vi "Outline_Station.vi"(8 "error in (no error)":errorcluster, 11 "Main":T1={"Tite"="", "Base path"=path "", "Table"=[], "Stations"=[], "Shield Array"=[], "UPHs"=[], "VISA"={"VISA"="", "baud rate"=9600, "data bits"=8, "parity"=enum."None", "stop bits"=10, "flow control"=0}, "Path"={"roof"=path "", "Config"=path "", "Png"=path ""}, "Ctr"={"DB Dispaly"=refnum, "Error Table"=refnum, "Display"=refnum, "Login"=refnum, "Exit"=refnum, "FTT_Submit"=refnum}, "Login"={"User"="", "Grade"=""}, "information"={"cause"="", "Type"=enum."Inform", "code"=0, "Suroce"="", "Status"=FALSE}, "Local DB"={"Connstr"="", "Database"={"Constr"={"Driver"="", "Server"="", "User"="", "Pwd"="", "Database"=""}, "conn ref"=refnum, "State"=FALSE}}, "Remote DB"={"Connstr"="", "Database"={"Constr"={"Driver"="", "Server"="", "User"="", "Pwd"="", "Database"=""}, "conn ref"=refnum, "State"=FALSE}}, "FTT TV"="", "ExchangeTime"=0, "NVH"="", "EOL Path"=path ""} {"VISA"."flow control" items=["None", "XON/XOFF", "RTS/CTS", "XON/XOFF & RTS/CTS", "DTR/DSR", "XON/XOFF & DTR/DSR"]; "VISA"."stop bits" items=["1.0"=10, "1.5"=15, "2.0"=20]}) -> (0 "error out":errorcluster)   [LabVIEW 2014]
uses:
  Type'def/Online_Table.ctl
  Simatic S7/Function/Read/Read Sigle Data/Read Sigle Bool.vi
  <vilib>/ptbypt/NI_PtbyPt.lvlib
  Simatic S7/Function/Read/Read Sigle Data/Read Sigle String.vi
  <vilib>/addons/database/_DB Variant To Data/Database Variant To Data.xnode
  Type'def/FTT Display Type.ctl
  Type'def/UPH Config.ctl
  VISA/Ctr/VISA Ctr.ctl
  Type'def/Main Ctr Ref.ctl
  Type'def/User Login.ctl
  Database/Ctr/Constr.ctl
  <vilib>/addons/database/Connection.llb/Conn ObjectReference.ctl
  <vilib>/addons/database/NI_Database_API.lvlib
  Database/Ctr/Conneect State.ctl
  Type'def/MainCtr.ctl
panel:
  in  "Boolean":bool
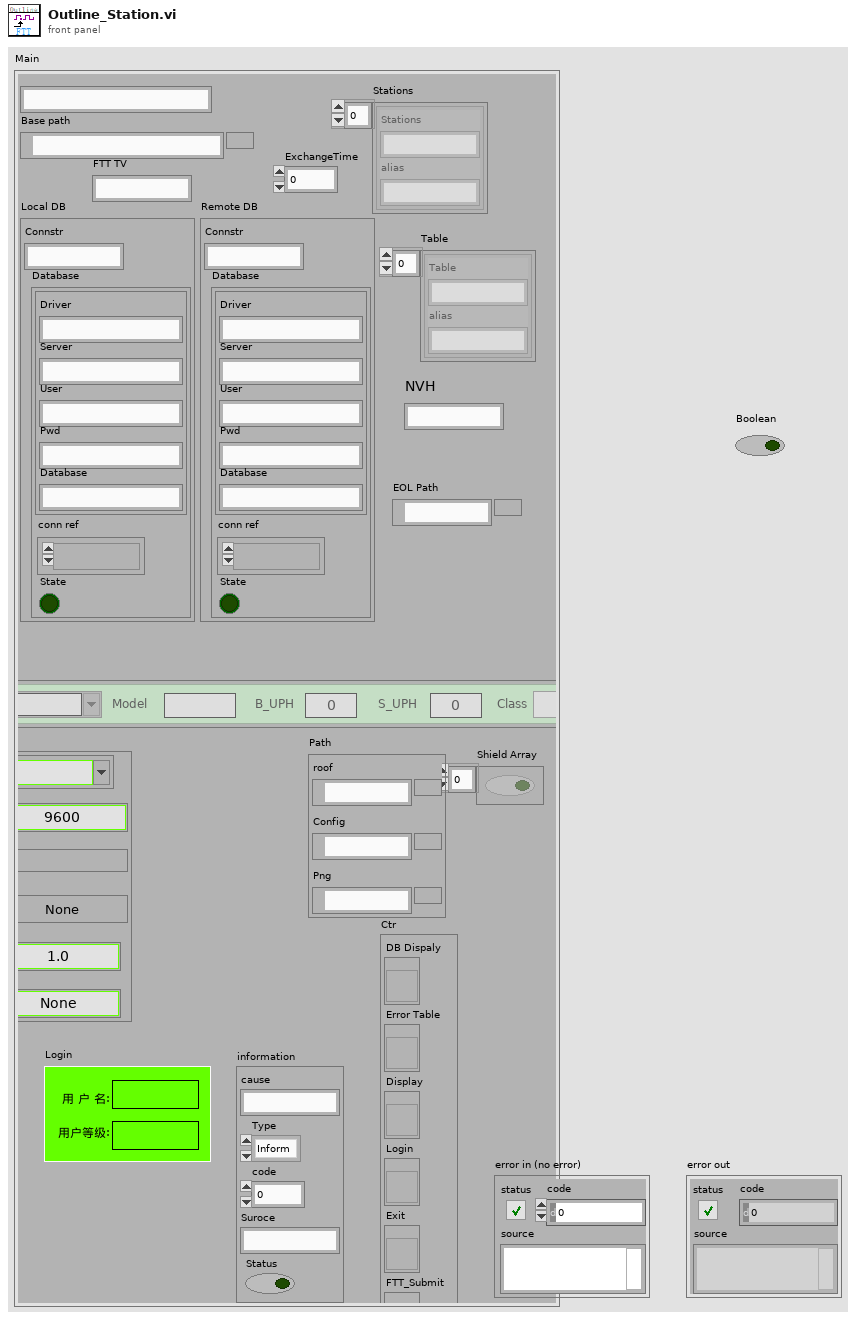
[diagram p1: front panel]
types:
  T1 = typedef "MainCtr.ctl" = cluster{"Tite":string, "Base path":path, "Table":cluster{"Table":string, "alias":string}[], "Stations":cluster{"Stations":string, "alias":string}[], "Shield Array":bool[], "UPHs":T2[], "VISA":T3, "Path":cluster{"roof":path, "Config":path, "Png":path}, "Ctr":T4, "Login":T5, "information":cluster{"cause":string, "Type":enum16{"Inform", "Warning", "Alarm"}, "code":i32, "Suroce":string, "Status":bool}, "Local DB":cluster{"Connstr":string, "Database":T6}, "Remote DB":cluster{"Connstr":string, "Database":T6}, "FTT TV":string, "ExchangeTime":i32, "NVH":string, "EOL Path":path}
  T2 = typedef "UPH Config.ctl" = cluster{"Line_No":string, "Model":string, "B_UPH ":i16, "S_UPH  ":i16, "Class":enum16{"Big", "Small"}}
  T3 = typedef "VISA Ctr.ctl" = cluster{"VISA":refnum<visa-resource-name>, "baud rate":u32, "data bits":u16, "parity":enum16{"None", "Odd", "Even", "Mark", "Space"}, "stop bits":u16, "flow control":u16}
  T4 = typedef "Main Ctr Ref.ctl" = cluster{"DB Dispaly":refnum<vi>, "Error Table":refnum<vi>, "Display":refnum<vi>, "Login":refnum<vi>, "Exit":refnum<vi>, "FTT_Submit":refnum<vi>}
  T5 = typedef "User Login.ctl" = cluster{"User":string, "Grade":string}
  T6 = typedef "Conneect State.ctl" = cluster{"Constr":T7, "conn ref":T8, "State":bool}
  T7 = typedef "Constr.ctl" = cluster{"Driver":string, "Server":string, "User":string, "Pwd":string, "Database":string}
  T8 = typedef "NI_Database_API.lvlib/Conn ObjectReference.ctl" = refnum<k1>
  T9 = typedef "FTT Display Type.ctl" = cluster{"Line.No":string, "Model":string, "Color":string, "UPH":dbl, "Plan":dbl, "Target Rate":dbl, "Target ":dbl, "Actual":dbl, "FTT":dbl, "FTT Rate":dbl, "Repaired":dbl, "Reject":dbl, "Ouline":dbl, "Line State":string}
  T10 = cluster{"cause":string, "Type":enum16{"Inform", "Warning", "Alarm"}, "code":i32, "Suroce":string, "Status":bool}
  T11 = typedef "Online_Table.ctl" = cluster{"SN":string, "Frame":string, "Station":string, "Model":string, "Color":string, "OnTime":timestamp, "OutTime":timestamp, "Repaired":i32, "OnRepair":bool, "Pstate":string}
  T12 = cluster{"Main ":T1, "Online_Table":T11, "information":cluster{"cause":string, "Type":enum16{"Inform", "Warning", "Alarm"}, "code":i32, "Suroce":string, "Status":bool}, "Display":T9}
  T13 = typedef "Phone Var.ctl" = cluster{"Mes":bool, "Model":string}
  T14 = cluster{"OutTime":timestamp, "Repaired":i32, "OnRepair":bool, "Pstate":string}
  T15 = cluster{"Display":T9, "Class":enum16{"Big", "Small"}}
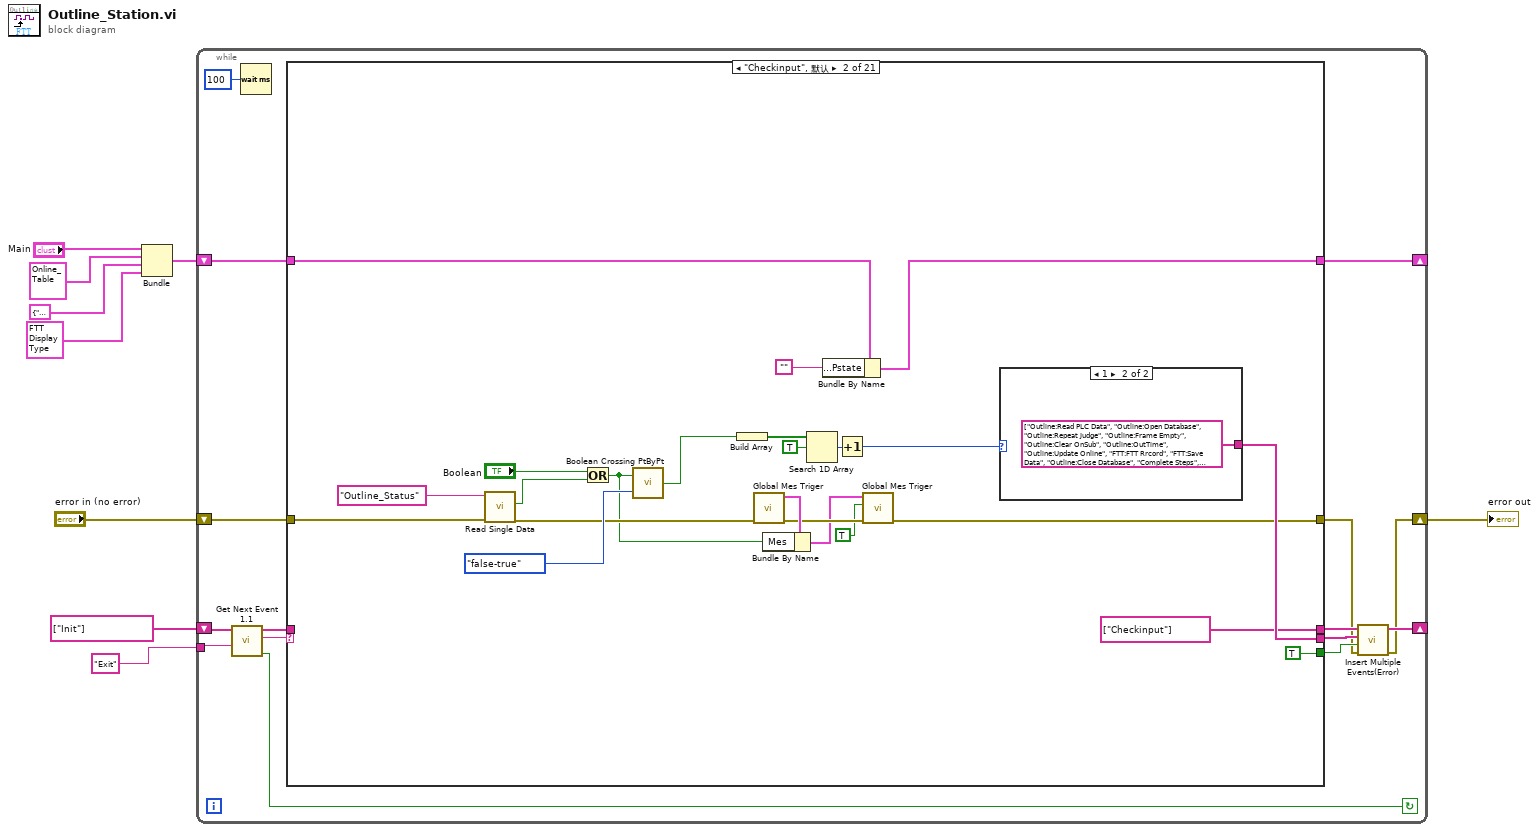
[diagram p0: block diagram]
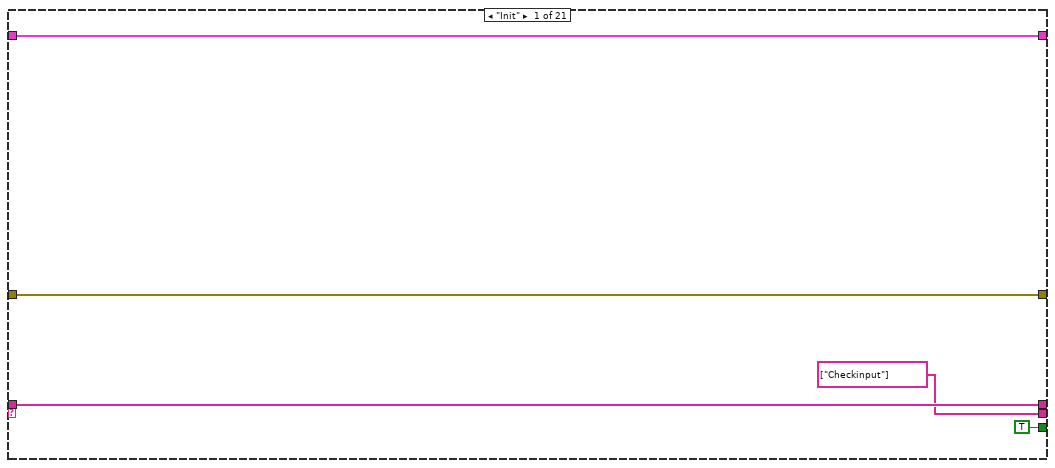
[diagram p2: hidden frame]
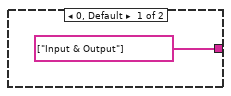
[diagram p3: hidden frame]
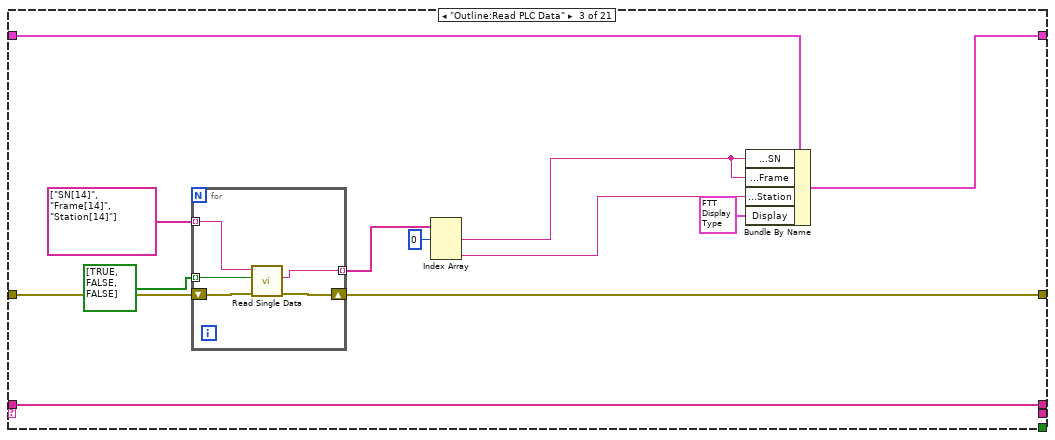
[diagram p4: hidden frame]
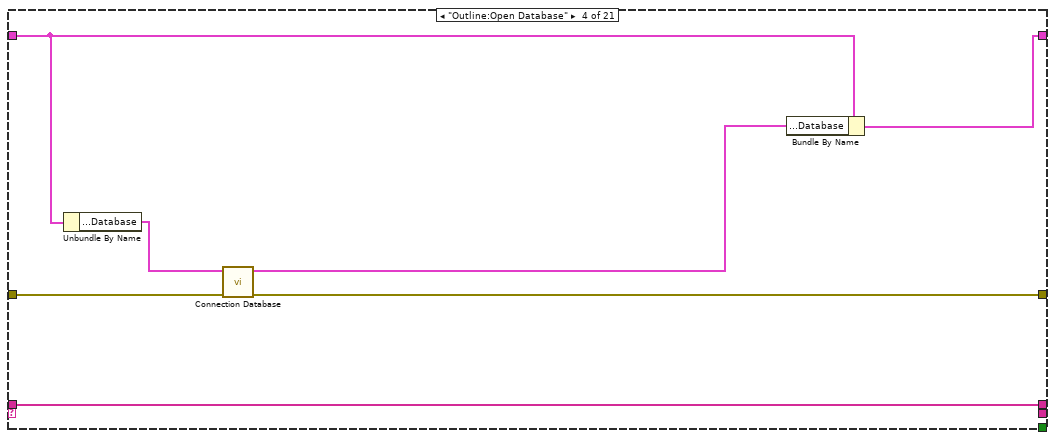
[diagram p5: hidden frame]
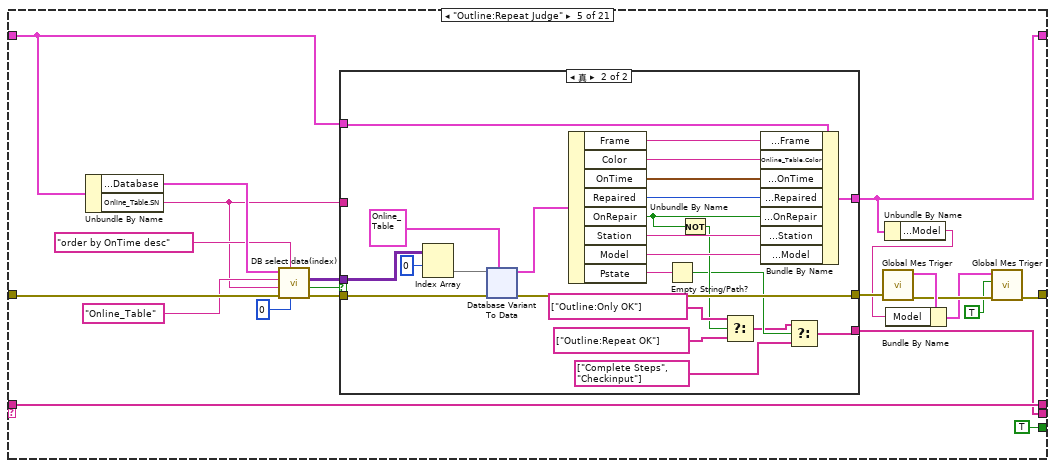
[diagram p6: hidden frame]
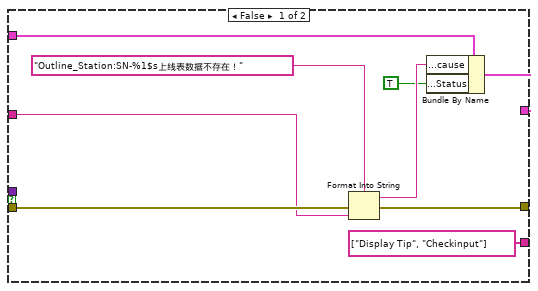
[diagram p7: hidden frame]
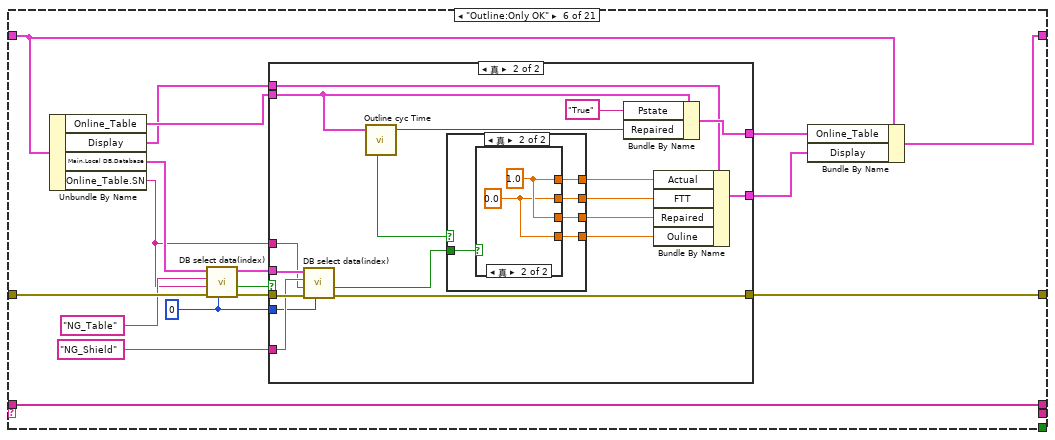
[diagram p8: hidden frame]
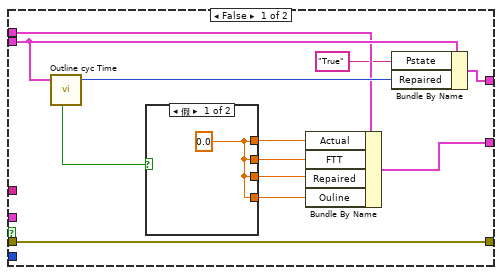
[diagram p9: hidden frame]
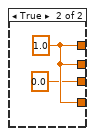
[diagram p10: hidden frame]
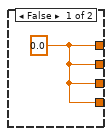
[diagram p11: hidden frame]
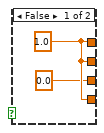
[diagram p12: hidden frame]
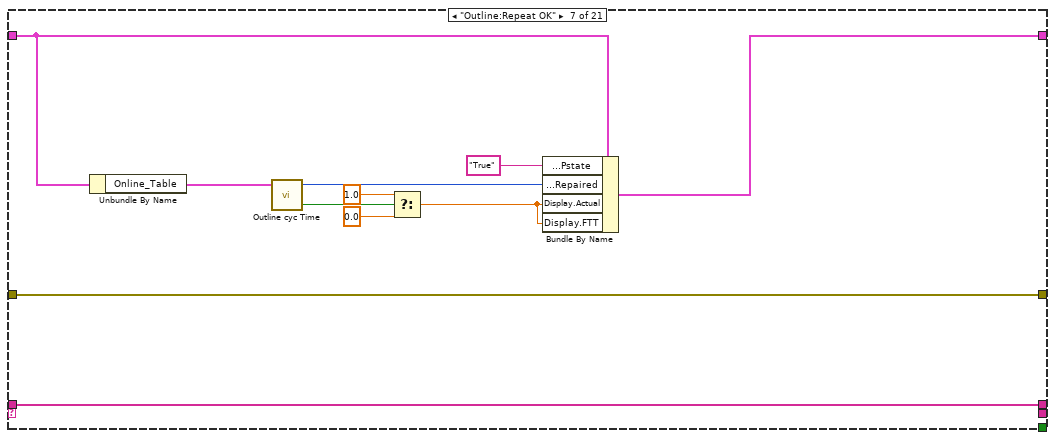
[diagram p13: hidden frame]
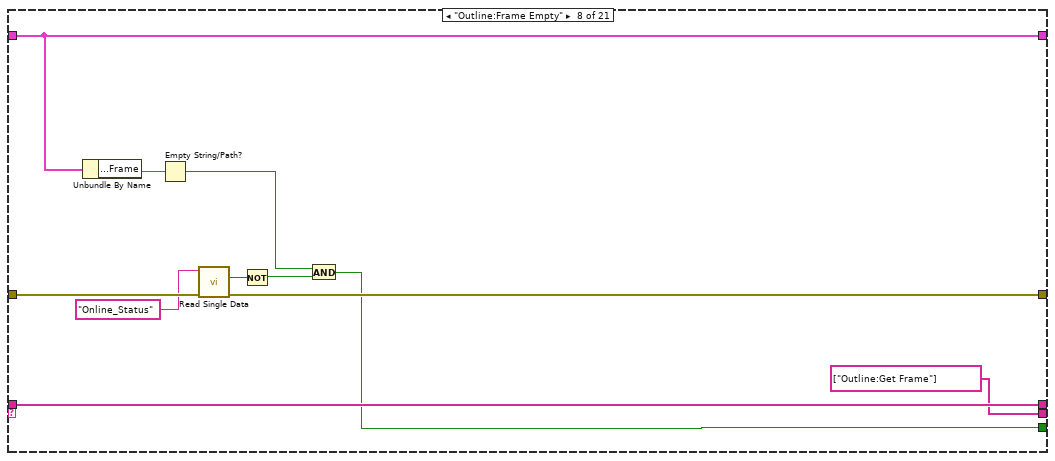
[diagram p14: hidden frame]
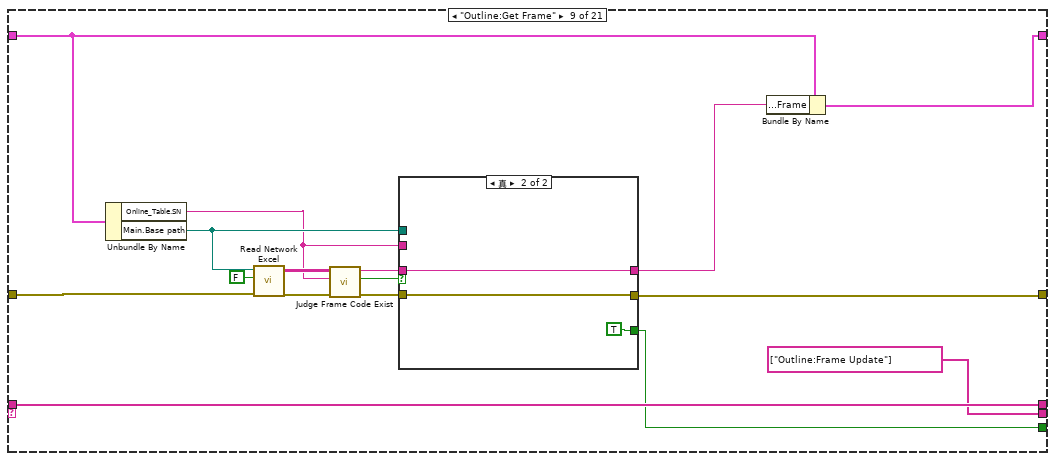
[diagram p15: hidden frame]
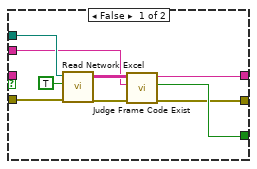
[diagram p16: hidden frame]
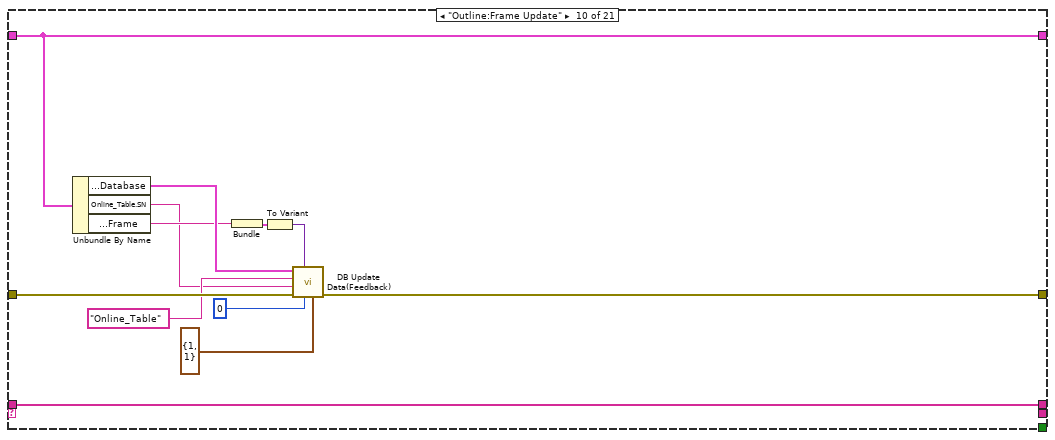
[diagram p17: hidden frame]
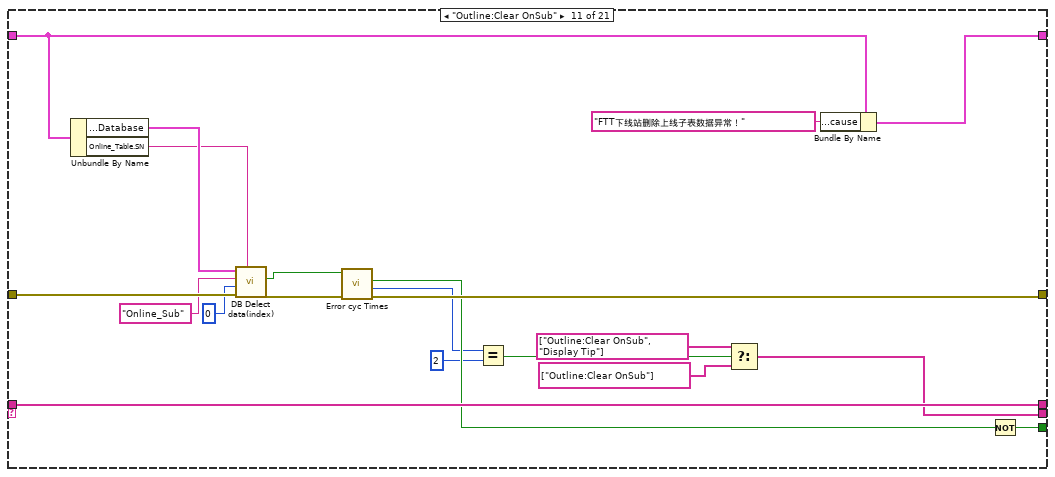
[diagram p18: hidden frame]
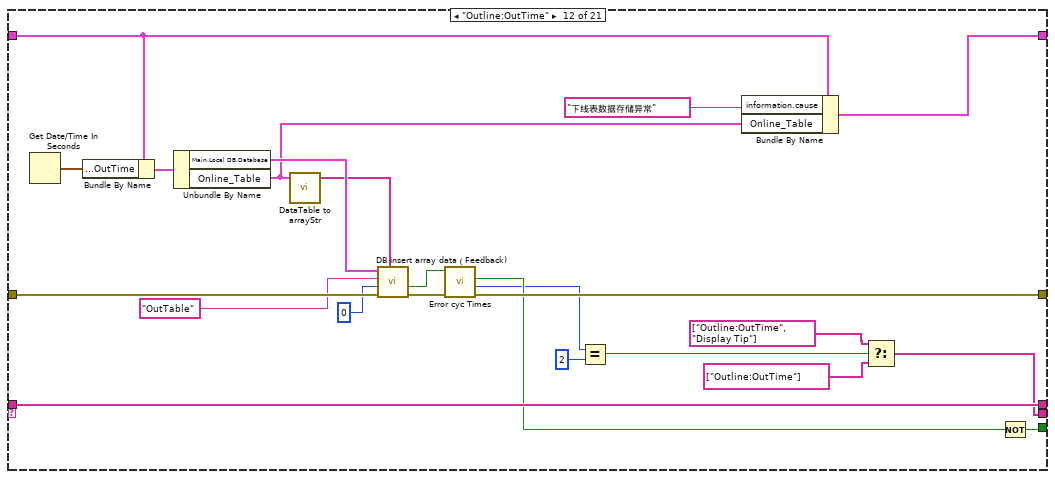
[diagram p19: hidden frame]
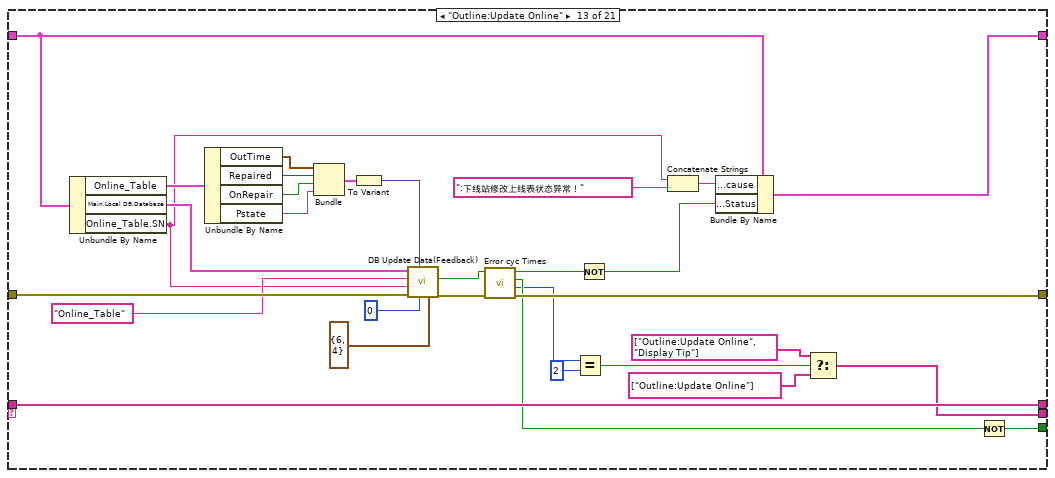
[diagram p20: hidden frame]
diagram:
  n1 = Bundle("Main"="Main", "Online_Table"=T11 {"SN"="", "Frame"="", "Station"="", "Model"="", "Color"="", "OnTime"=timestamp(0 s since 1904-01-01), "OutTime"=timestamp(0 s since 1904-01-01), "Repaired"=0, "OnRepair"=FALSE, "Pstate"=""}, "information"=T10 {"cause"="", "Type"=enum."Inform", "code"=0, "Suroce"="", "Status"=FALSE}, "Display"=T9 {"Line.No"="", "Model"="", "Color"="", "UPH"=0.0, "Plan"=0.0, "Target Rate"=0.0, "Target "=0.0, "Actual"=0.0, "FTT"=0.0, "FTT Rate"=0.0, "Repaired"=0.0, "Reject"=0.0, "Ouline"=0.0, "Line State"=""}) -> (w6:T12)  [unwired: 1 in]
  n2 = while {
    tunnel: "Exit" ("Exit Event") -> [w21]
    shift-right: [w17] -> _
    shift-left: string[] ["Init"] -> [w22]
    shift-right: [w10] -> w3
    shift-left: "error in (no error)" -> [w20]
    shift-right: [w13] -> _
    shift-left: w6 -> [w18]
    stop <- w23 continue-if-true
    n3 = call "Get Next Event 1.1.vi"("Exit Event"=w21, "event queue in"=w22) -> ("Condition (Exit:F)"=w23:bool, "next event"=w24:string, "event queue out"=w19:string[])  [unwired: 6 in, 1 out]
    n4 = Wait (ms)(milliseconds to wait=u32 100) -> ()  [unwired: 1 out]
    n5 = case shown="\"Checkinput\", 默认" w24 {
      tunnel: w20 -> [w27 w50 w64 w77 w99 w489 w543 w551 w562 w592 w613 w635 w668 w675 w702 w729 w754 w759 w765 w768 w776]
      tunnel: w19 -> [w29 _ w62 w72 w92 w487 w542 w552 w560 w594 w614 w637 w658 w670 w701 w721 w753 w760 w764 w771 w779]
      tunnel: w18 -> [w28 w41 w66 w75 w90 w481 w539 w553 w559 w593 w597 w618 w648 w673 w679 w719 w749 w761 w766 w772 w783]
      tunnel: [w27 w30 w63 w76 w81 w476 w543 w549 w561 w588 w606 w627 w653 w671 w680 w715 w754 w755 w765 w773 w784] -> w11
      tunnel: [w29 string[] ["Checkinput"] w62 w72 w92 w487 w542 w552 w560 w594 w614 w637 w658 w670 w701 w721 w753 w760 w764 w771 w779] -> w16
      tunnel: [TRUE ("Insert all? (T)") TRUE ("Insert all? (T)") _ _ TRUE ("Insert all? (T)") _ _ w545 w555 _ w605 w626 w652 _ _ w714 _ w757 TRUE ("Insert all? (T)") _ TRUE ("Insert all? (T)")] -> w15
      tunnel: [string[] ["Checkinput"] w51 _ _ w89 _ _ string[] ["Outline:Get Frame"] string[] ["Outline:Frame Update"] _ w599 w619 w641 _ _ w709 _ string[] ["Quit"] string[] ["Exit"] _ string[] ["Checkinput"]] -> w14
      tunnel: [w28 w40 w65 w78 w80 w480 w538 w553 w557 w593 w596 w617 w647 w669 w678 w718 w748 w761 w766 w772 w783] -> w13
      frame "Init" {
      }
      frame "Checkinput", Default {
        n6 = call-poly "Read Single Data.vi"("error in (no error)"=w50, "Tags"="Outline_Status") -> ("error out"=w37:errorcluster, "Boolean"=w48:bool)  [unwired: 7 in, 1 out]
        n7 = Or(x="Boolean", y=w48) -> (x .or. y?=w34:bool)
        n8 = call <vilib>:"Boolean Crossing PtByPt.vi"("direction"=enum16{"either", "false-true", "true-false"}."false-true", "input"=w34) -> ("crossing"=w36:bool)  [unwired: 1 in]
        n9 = Build Array(w36) -> (w46:bool[])
        n10 = call "Global Mes Triger.vi"("error in (no error)"=w37) -> ("error out"=w33:errorcluster, "Var out"=w35:T13)  [unwired: 9 in]
        n11 = Bundle By Name(cluster=w35, "Mes"=w34) -> (w32:T13)
        n12 = Search 1D Array(1D array=w46, element=TRUE) -> (index of element=w44:i32)  [unwired: 1 in]
        n13 = Bundle By Name(cluster=w41, "Online_Table.Pstate"="") -> (w40:T12)
        n14 = Increment(x=w44) -> (x+1=w43:i32)
        n15 = call "Global Mes Triger.vi"("error in (no error)"=w33, "R/S"=TRUE, "Var"=w32) -> ("error out"=w30:errorcluster)  [unwired: 7 in, 1 out]
        n16 = case shown="1" w43 {
          tunnel: [string[] ["Input & Output"] string[] ["Outline:Read PLC Data", "Outline:Open Database", "Outline:Repeat Judge", "Outline:Frame Empty", "Outline:Clear OnSub", "Outline:OutTime", "Outline:Update Online", "FTT:FTT Rrcord", "FTT:Save Data", "Outline:Close Database", "Complete Steps", "Display Tip", "Checkinput"]] -> w51
          frame 0, Default {
          }
          frame 1 {
          }
        }
      }
      frame "Outline:Read PLC Data" {
        n17 = for {
          shift-right: [w70] -> w63
          shift-left: w64 -> [w71]
          tunnel: string[] ["SN[14]", "Frame[14]", "Station[14]"] -> [w69] mode=indexing
          tunnel: [w68] -> w60 mode=indexing
          tunnel: bool[] [TRUE, FALSE, FALSE] -> [w67] mode=indexing
          n18 = call-poly "Read Single Data.vi"("error in (no error)"=w71, "Char/Str"=w67, "Tags"=w69) -> ("error out"=w70:errorcluster, "Data Byte"=w68:string)  [unwired: 6 in, 1 out]
        }
        n19 = Index Array(array=w60, index #1=0 ("index")) -> (element #1=w56:string, element #3=w58:string)  [unwired: 2 in, 1 out]
        n20 = Bundle By Name(cluster=w66, "Online_Table.SN"=w56, "Online_Table.Frame"=w56, "Online_Table.Station"=w58, "Display"=T9 {"Line.No"="", "Model"="", "Color"="", "UPH"=0.0, "Plan"=0.0, "Target Rate"=0.0, "Target "=0.0, "Actual"=0.0, "FTT"=0.0, "FTT Rate"=0.0, "Repaired"=0.0, "Reject"=0.0, "Ouline"=0.0, "Line State"=""}) -> (w65:T12)
      }
      frame "Outline:Open Database" {
        n21 = Unbundle By Name(w75) -> ("Main.Local DB.Database"=w74:T6)
        n22 = call "Connection Database.vi"("error in (no error)"=w77, "Connncet State"=w74) -> ("error out"=w76:errorcluster, "Connncet State out"=w73:T6)  [unwired: 8 in]
        n23 = Bundle By Name(cluster=w75, "Main.Local DB.Database"=w73) -> (w78:T12)
      }
      frame "Outline:Repeat Judge" {
        n24 = Unbundle By Name(w90) -> ("Main.Local DB.Database"=w98:T6, "Online_Table.SN"=w87:string)
        n25 = call "DB select data(index).vi"("index"=0, "Condtion"="order by OnTime desc", "error in (no error)"=w99, "Code"=w87, "Tabe"="Online_Table", "Connncet State"=w98) -> ("error out"=w93:errorcluster, "state"=w88:bool, "data"=w94:variant[][])  [unwired: 2 in, 1 out]
        n26 = case shown="真" w88 {
          tunnel: w94 -> [_ w132]
          tunnel: w93 -> [w105 w130]
          tunnel: [w104 w122] -> w82
          tunnel: w90 -> [w107 w121]
          tunnel: [w106 w120] -> w80
          tunnel: [string[] ["Display Tip", "Checkinput"] w111] -> w89
          tunnel: w87 -> [w102 _]
          frame False {
            n27 = Format Into String(format string="Outline_Station:SN-%1$s上线表数据不存在！", error in=w105, w102) -> (resulting string=w101:string, error out=w104:errorcluster)  [unwired: 1 in]
            n28 = Bundle By Name(cluster=w107, "information.cause"=w101, "information.Status"=TRUE) -> (w106:T12)
          }
          frame True {
            n29 = Index Array(array=w132, index (row)=0) -> (element=w129:variant[])  [unwired: 1 in]
            n30 = xnode "Database Variant To Data"("database variant"=w129, "error in (no error)"=w130, "type"=T11 {"SN"="", "Frame"="", "Station"="", "Model"="", "Color"="", "OnTime"=timestamp(0 s since 1904-01-01), "OutTime"=timestamp(0 s since 1904-01-01), "Repaired"=0, "OnRepair"=FALSE, "Pstate"=""} ("Online_Table")) -> ("data"=w127:T11, "error out"=w122:errorcluster)
            n31 = Unbundle By Name(w127) -> ("Frame"=w126:string, "Color"=w125:string, "OnTime"=w124:timestamp, "Repaired"=w123:i32, "OnRepair"=w115:bool, "Station"=w117:string, "Model"=w116:string, "Pstate"=w113:string)
            n32 = Empty String/Path?(string/path=w113) -> (empty?=w112:bool)
            n33 = Not(x=w115) -> (.not. x?=w114:bool)
            n34 = Select(t=string[] ["Outline:Only OK"], s=w114, f=string[] ["Outline:Repeat OK"]) -> (s? t:f=w110:string[])
            n35 = Bundle By Name(cluster=w121, "Online_Table.Frame"=w126, "Online_Table.Color"=w125, "Online_Table.OnTime"=w124, "Online_Table.Repaired"=w123, "Online_Table.OnRepair"=w115, "Online_Table.Station"=w117, "Online_Table.Model"=w116) -> (w120:T12)
            n36 = Select(t=w110, s=w112, f=string[] ["Complete Steps", "Checkinput"]) -> (s? t:f=w111:string[])
          }
        }
        n37 = call "Global Mes Triger.vi"("error in (no error)"=w82) -> ("error out"=w85:errorcluster, "Var out"=w86:T13)  [unwired: 9 in]
        n38 = Unbundle By Name(w80) -> ("Online_Table.Model"=w79:string)
        n39 = Bundle By Name(cluster=w86, "Model"=w79) -> (w84:T13)
        n40 = call "Global Mes Triger.vi"("error in (no error)"=w85, "R/S"=TRUE, "Var"=w84) -> ("error out"=w81:errorcluster)  [unwired: 7 in, 1 out]
      }
      frame "Outline:Only OK" {
        w473 = 0 ("index")
        n41 = Unbundle By Name(w481) -> ("Online_Table"=w478:T11, "Display"=w477:T9, "Main.Local DB.Database"=w488:T6, "Online_Table.SN"=w474:string)
        n42 = call "DB select data(index).vi"("index"=w473, "error in (no error)"=w489, "Code"=w474, "Tabe"="NG_Table", "Connncet State"=w488) -> ("error out"=w486:errorcluster, "state"=w485:bool, "Connncet State out"=w483:T6)  [unwired: 3 in, 1 out]
        n43 = case shown="真" w485 {
          tunnel: w486 -> [w496 w520]
          tunnel: w478 -> [w499 w506]
          tunnel: w483 -> [_ w519]
          tunnel: "NG_Shield" -> [_ w518]
          tunnel: [w500 w522] -> w479
          tunnel: w477 -> [w497 w514]
          tunnel: [w496 w516] -> w476
          tunnel: [w495 w513] -> w475
          tunnel: w474 -> [_ w517]
          tunnel: w473 -> [_ w507]
          frame False {
            n44 = call "Outline cyc Time.vi"("Online_Table"=w499) -> ("Pstates"=w498:bool, "Repair"=w501:i32)  [unwired: 7 in]
            n45 = case shown="假" w498 {
              tunnel: [w502 w504] -> w494
              tunnel: [w502 w504] -> w493
              tunnel: [w502 w504] -> w492
              tunnel: [w502 0.0] -> w491
              frame False {
                w502 = 0.0
              }
              frame True {
                w504 = 1.0
              }
            }
            n46 = Bundle By Name(cluster=w497, "Actual"=w494, "FTT"=w493, "Repaired"=w491, "Ouline"=w492) -> (w495:T9)
            n47 = Bundle By Name(cluster=w499, "Pstate"="True", "Repaired"=w501) -> (w500:T11)
          }
          frame True {
            n48 = call "DB select data(index).vi"("index"=w507, "error in (no error)"=w520, "Code"=w517, "Tabe"=w518, "Connncet State"=w519) -> ("error out"=w516:errorcluster, "state"=w508:bool)  [unwired: 3 in, 2 out]
            n49 = call "Outline cyc Time.vi"("Online_Table"=w506) -> ("Pstates"=w515:bool, "Repair"=w521:i32)  [unwired: 7 in]
            n50 = case shown="真" w515 {
              tunnel: [w523 w527] -> w512
              tunnel: [w523 w526] -> w511
              tunnel: [w523 w525] -> w510
              tunnel: [w523 w524] -> w509
              tunnel: w508 -> [_ w528]
              frame False {
                w523 = 0.0
              }
              frame True {
                n51 = case shown="真" w528 {
                  tunnel: [w530 w532] -> w527
                  tunnel: [w530 w531] -> w526
                  tunnel: [0.0 w532] -> w525
                  tunnel: [w530 w531] -> w524
                  frame False {
                    w530 = 1.0
                  }
                  frame True {
                    w531 = 0.0
                    w532 = 1.0
                  }
                }
              }
            }
            n52 = Bundle By Name(cluster=w506, "Pstate"="True", "Repaired"=w521) -> (w522:T11)
            n53 = Bundle By Name(cluster=w514, "Actual"=w512, "FTT"=w511, "Repaired"=w510, "Ouline"=w509) -> (w513:T9)
          }
        }
        n54 = Bundle By Name(cluster=w481, "Online_Table"=w479, "Display"=w475) -> (w480:T12)
      }
      frame "Outline:Repeat OK" {
        n55 = Unbundle By Name(w539) -> ("Online_Table"=w541:T11)
        n56 = call "Outline cyc Time.vi"("Online_Table"=w541) -> ("Pstates"=w537:bool, "Repair"=w540:i32)  [unwired: 7 in]
        n57 = Select(t=1.0, s=w537, f=0.0) -> (s? t:f=w533:dbl)
        n58 = Bundle By Name(cluster=w539, "Online_Table.Pstate"="True", "Online_Table.Repaired"=w540, "Display.Actual"=w533, "Display.FTT"=w533) -> (w538:T12)
      }
      frame "Outline:Frame Empty" {
        n59 = Unbundle By Name(w553) -> ("Online_Table.Frame"=w554:string)
        n60 = Empty String/Path?(string/path=w554) -> (empty?=w546:bool)
        n61 = call-poly "Read Single Data.vi"("error in (no error)"=w551, "Tags"="Online_Status") -> ("error out"=w549:errorcluster, "Boolean"=w548:bool)  [unwired: 7 in, 1 out]
        n62 = Not(x=w548) -> (.not. x?=w547:bool)
        n63 = And(x=w546, y=w547) -> (x .and. y?=w545:bool)
      }
      frame "Outline:Get Frame" {
        n64 = Unbundle By Name(w559) -> ("Online_Table.SN"=w564:string, "Main.Base path"=w565:path)
        n65 = call "Read Network Excel.vi"("error in (no error)"=w562, "T/Y"=FALSE, "Base Path"=w565) -> ("error out"=w570:errorcluster, "2DA_Str"=w569:string[][])  [unwired: 7 in]
        n66 = call "Judge Frame Code Exist.vi"("error in (no error)"=w570, "Online_Table.SN"=w564, "2DA_Str"=w569) -> ("error out"=w568:errorcluster, "Status"=w567:bool, "Frame Code"=w566:string)  [unwired: 6 in]
        n67 = case shown="真" w567 {
          tunnel: w568 -> [w578 w580]
          tunnel: w566 -> [_ w582]
          tunnel: [w572 w582] -> w558
          tunnel: w565 -> [w577 _]
          tunnel: w564 -> [w574 _]
          tunnel: [w573 TRUE ("Status")] -> w555
          tunnel: [w571 w580] -> w561
          frame False {
            n68 = call "Read Network Excel.vi"("error in (no error)"=w578, "T/Y"=TRUE, "Base Path"=w577) -> ("error out"=w579:errorcluster, "2DA_Str"=w575:string[][])  [unwired: 7 in]
            n69 = call "Judge Frame Code Exist.vi"("error in (no error)"=w579, "Online_Table.SN"=w574, "2DA_Str"=w575) -> ("error out"=w571:errorcluster, "Status"=w573:bool, "Frame Code"=w572:string)  [unwired: 6 in]
          }
          frame True {
          }
        }
        n70 = Bundle By Name(cluster=w559, "Online_Table.Frame"=w558) -> (w557:T12)
      }
      frame "Outline:Frame Update" {
        n71 = Unbundle By Name(w593) -> ("Main.Local DB.Database"=w591:T6, "Online_Table.SN"=w583:string, "Online_Table.Frame"=w587:string)
        n72 = Bundle("Frame"=w587) -> (w586:cluster{"Frame":string})  [unwired: 1 in]
        n73 = To Variant(anything=w586) -> (Variant=w585:variant)
        n74 = call "DB Update Data(Feedback).vi"("Pos"=cluster{"index":i32, "Len":i32} {"index"=1, "Len"=1}, "Sel index"=0, "data"=w585, "error in (no error)"=w592, "Code"=w583, "table"="Online_Table", "Connncet State"=w591) -> ("error out"=w588:errorcluster)  [unwired: 2 in, 2 out]
      }
      frame "Outline:Clear OnSub" {
        n75 = Unbundle By Name(w597) -> ("Main.Local DB.Database"=w612:T6, "Online_Table.SN"=w610:string)
        n76 = call "DB Delect data(index).vi"("code"=w610, "error in (no error)"=w613, "index"=0, "table"="Online_Sub", "Connncet State"=w612) -> ("error out"=w608:errorcluster, "Boolean"=w607:bool)  [unwired: 4 in, 1 out]
        n77 = call "Error cyc Times.vi"("error in (no error)"=w608, "Status in"=w607) -> ("error out"=w606:errorcluster, "Numeric"=w603:i32, "Cys Status"=w604:bool)  [unwired: 6 in, 1 out]
        n78 = Equal?(x=w603, y=2) -> (x = y?=w601:bool)
        n79 = Select(t=string[] ["Outline:Clear OnSub", "Display Tip"], s=w601, f=string[] ["Outline:Clear OnSub"]) -> (s? t:f=w599:string[])
        n80 = Bundle By Name(cluster=w597, "information.cause"="FTT下线站删除上线子表数据异常！") -> (w596:T12)
        n81 = Not(x=w604) -> (.not. x?=w605:bool)
      }
      frame "Outline:OutTime" {
        n82 = Get Date/Time In Seconds() -> (seconds since 1Jan1904=w636:timestamp)
        n83 = Bundle By Name(cluster=w618, "Online_Table.OutTime"=w636) -> (w631:T12)
        n84 = Unbundle By Name(w631) -> ("Main.Local DB.Database"=w632:T6, "Online_Table"=w615:T11)
        n85 = call "DataTable to arrayStr.vi"("Online_Table"=w615) -> ("appended array"=w630:string[])  [unwired: 4 in]
        n86 = call "DB insert array data（Feedback).vi"("Data"=w630, "error in (no error)"=w635, "index"=0, "table"="OutTable", "Connncet State"=w632) -> ("error out"=w629:errorcluster, "state"=w628:bool)  [unwired: 4 in, 1 out]
        n87 = call "Error cyc Times.vi"("error in (no error)"=w629, "Status in"=w628) -> ("error out"=w627:errorcluster, "Numeric"=w624:i32, "Cys Status"=w625:bool)  [unwired: 6 in, 1 out]
        n88 = Equal?(x=w624, y=2) -> (x = y?=w622:bool)
        n89 = Bundle By Name(cluster=w618, "information.cause"="下线表数据存储异常", "Online_Table"=w615) -> (w617:T12)
        n90 = Select(t=string[] ["Outline:OutTime", "Display Tip"], s=w622, f=string[] ["Outline:OutTime"]) -> (s? t:f=w619:string[])
        n91 = Not(x=w625) -> (.not. x?=w626:bool)
      }
      frame "Outline:Update Online" {
        n92 = Unbundle By Name(w648) -> ("Online_Table"=w663:T11, "Main.Local DB.Database"=w667:T6, "Online_Table.SN"=w638:string)
        n93 = Unbundle By Name(w663) -> ("OutTime"=w662:timestamp, "Repaired"=w661:i32, "OnRepair"=w660:bool, "Pstate"=w659:string)
        n94 = Bundle("OutTime"=w662, "Repaired"=w661, "OnRepair"=w660, "Pstate"=w659) -> (w657:T14)  [unwired: 1 in]
        n95 = To Variant(anything=w657) -> (Variant=w656:variant)
        n96 = call "DB Update Data(Feedback).vi"("Pos"=cluster{"index":i32, "Len":i32} {"index"=6, "Len"=4}, "Sel index"=0, "data"=w656, "error in (no error)"=w668, "Code"=w638, "table"="Online_Table", "Connncet State"=w667) -> ("error out"=w655:errorcluster, "State"=w654:bool)  [unwired: 2 in, 1 out]
        n97 = call "Error cyc Times.vi"("error in (no error)"=w655, "Status in"=w654) -> ("error out"=w653:errorcluster, "Numeric"=w646:i32, "Cys Status"=w651:bool, "Status out"=w650:bool)  [unwired: 6 in]
        n98 = Equal?(x=w646, y=2) -> (x = y?=w644:bool)
        n99 = Not(x=w650) -> (.not. x?=w649:bool)
        n100 = Concatenate Strings(w638, ":下线站修改上线表状态异常！" ("information.cause")) -> (w640:string)
        n101 = Bundle By Name(cluster=w648, "information.cause"=w640, "information.Status"=w649) -> (w647:T12)
        n102 = Select(t=string[] ["Outline:Update Online", "Display Tip"], s=w644, f=string[] ["Outline:Update Online"]) -> (s? t:f=w641:string[])
        n103 = Not(x=w651) -> (.not. x?=w652:bool)
      }
      frame "Outline:Close Database" {
        n104 = Unbundle By Name(w673) -> ("Main.Local DB.Database"=w674:T6)
        n105 = call "Disconncetion DB.vi"("error in (no error)"=w675, "Connncet State"=w674) -> ("error out"=w671:errorcluster, "Connect State"=w672:T6)  [unwired: 8 in]
        n106 = Bundle By Name(cluster=w673, "Main.Local DB.Database"=w672) -> (w669:T12)
      }
      frame "FTT:FTT Rrcord" {
        n107 = call "Global FTT Data.vi"("error in (no error)"=w702, "Mode"=enum16{"Read", "Write"}."Read") -> ("error out"=w683:errorcluster, "Cluster"=w699:T15)  [unwired: 8 in]
        n108 = Unbundle By Name(w699) -> ("Display.Actual"=w697:dbl, "Display.FTT"=w694:dbl, "Display.Repaired"=w691:dbl, "Display.Reject"=w688:dbl, "Display.Ouline"=w685:dbl)
        n109 = Unbundle By Name(w679) -> ("Display.Actual"=w696:dbl, "Display.FTT"=w693:dbl, "Display.Repaired"=w690:dbl, "Display.Reject"=w687:dbl, "Display.Ouline"=w684:dbl)
        n110 = Add(x=w684, y=w685) -> (x+y=w686:dbl)
        n111 = Add(x=w687, y=w688) -> (x+y=w689:dbl)
        n112 = Add(x=w690, y=w691) -> (x+y=w692:dbl)
        n113 = Add(x=w693, y=w694) -> (x+y=w695:dbl)
        n114 = Add(x=w696, y=w697) -> (x+y=w698:dbl)
        n115 = Bundle By Name(cluster=w699, "Display.Actual"=w698, "Display.FTT"=w695, "Display.Repaired"=w692, "Display.Reject"=w689, "Display.Ouline"=w686) -> (w681:T15)
        n116 = call "Global FTT Data.vi"("error in (no error)"=w683, "Mode"=enum16{"Read", "Write"}."Write", "Display"=w681) -> ("error out"=w680:errorcluster, "Cluster"=w677:T15)  [unwired: 7 in]
        n117 = Unbundle By Name(w677) -> ("Display"=w676:T9)
        n118 = Bundle By Name(cluster=w679, "Display"=w676) -> (w678:T12)
      }
      frame "FTT:Save Data" {
        w722 = "[FTT_Clinet].[dbo].[FTT1_ Write]"
        n119 = Unbundle By Name(w719) -> ("Online_Table.SN"=w704:string, "Main.Local DB.Database"=w728:T6, "Display.Line.No"=w720:string, "Display"=w724:T9)
        n120 = call "DB select data(index).vi"("index"=0, "error in (no error)"=w729, "Code"=w720, "Tabe"=w722, "Connncet State"=w728) -> ("error out"=w726:errorcluster, "state"=w725:bool, "Connncet State out"=w723:T6)  [unwired: 3 in, 1 out]
        n121 = case shown="真" w725 {
          tunnel: w726 -> [w737 w746]
          tunnel: w724 -> [w736 w744]
          tunnel: w723 -> [w734 w745]
          tunnel: w722 -> [w733 w741]
          tunnel: [w731 w739] -> w717
          tunnel: w720 -> [_ w740]
          tunnel: [w730 w738] -> w716
          frame False {
            n122 = call "ftt array.vi"("Display"=w736) -> ("appended array"=w735:string[])  [unwired: 4 in]
            n123 = call "DB insert array data（Feedback).vi"("Data"=w735, "error in (no error)"=w737, "index"=0, "table"=w733, "Connncet State"=w734) -> ("error out"=w731:errorcluster, "state"=w730:bool)  [unwired: 4 in, 1 out]
          }
          frame True {
            n124 = call "DB Update Data(Feedback).vi"("Pos"=cluster{"index":i32, "Len":i32} {"index"=0, "Len"=14}, "Sel index"=0, "data"=w744, "error in (no error)"=w746, "Code"=w740, "table"=w741, "Connncet State"=w745) -> ("error out"=w739:errorcluster, "State"=w738:bool)  [unwired: 2 in, 1 out]
          }
        }
        n125 = call "Error cyc Times.vi"("error in (no error)"=w717, "Status in"=w716) -> ("error out"=w715:errorcluster, "Numeric"=w712:i32, "Cys Status"=w713:bool)  [unwired: 6 in, 1 out]
        n126 = Equal?(x=w712, y=2) -> (x = y?=w710:bool)
        n127 = Concatenate Strings("下线站SN:" ("information.cause"), w704, "修改FTT数据表异常") -> (w706:string)
        n128 = Select(t=string[] ["FTT:Save Data", "Display Tip"], s=w710, f=string[] ["FTT:Save Data"]) -> (s? t:f=w709:string[])
        n129 = Bundle By Name(cluster=w719, "information.cause"=w706) -> (w718:T12)
        n130 = Not(x=w713) -> (.not. x?=w714:bool)
      }
      frame "Complete Steps" {
        n131 = Unbundle By Name(w749) -> ("Online_Table.SN"=w751:string)
        n132 = Concatenate Strings(w751, ":天窗下线完成!" ("string")) -> (w752:string)
        n133 = Bundle By Name(cluster=w749, "information.cause"=w752, "Online_Table"=T11 {"SN"="", "Frame"="", "Station"="", "Model"="", "Color"="", "OnTime"=timestamp(0 s since 1904-01-01), "OutTime"=timestamp(0 s since 1904-01-01), "Repaired"=0, "OnRepair"=FALSE, "Pstate"=""}) -> (w748:T12)
      }
      frame "Input & Output" {
        n134 = Unbundle By Name(w761) -> ("Main.Ctr.Exit"=w758:refnum<vi>)
        n135 = property class="Bool (严格)"(reference=w758, error in=w759) -> (error out=w755:errorcluster, "Value"=w757:bool)  [unwired: 1 out]
      }
      frame "Quit" {
      }
      frame "Display Tip" {
        n136 = Unbundle By Name(w772) -> ("information"=w770:T10)
        n137 = Unbundle By Name(w768) -> ("source"=w767:string)
        n138 = Bundle By Name(cluster=w770, "Suroce"=w767) -> (w769:T10)
        n139 = call "Log info.vi"("error in (no error)"=w768, "information"=w769) -> ("error out"=w773:errorcluster)  [unwired: 8 in, 1 out]
      }
      frame "Error Log" {
        n140 = Unbundle By Name(w783) -> ("information"=w782:T10)
        n141 = Unbundle By Name(w776) -> ("source"=w775:string, "status"=w774:bool)
        n142 = Bundle By Name(cluster=w782, "Status"=TRUE, "Suroce"=w775, "Status"=w774) -> (w781:T10)
        n143 = call "Log info.vi"("error in (no error)"=w776, "information"=w781) -> ("error out"=w785:errorcluster)  [unwired: 8 in, 1 out]
        n144 = call <vilib>:"Clear Errors.vi"("error in (no error)"=w785) -> ("error out"=w784:errorcluster)  [unwired: 5 in, 1 out]
      }
    }
    n145 = call "Insert Multiple Events(Error).vi"("error in (no error)"=w11, "Insert all? (T)"=w15, "Events to Insert"=w14, "Event queue in"=w16) -> ("error out"=w10:errorcluster, "Event queue out"=w17:string[])  [unwired: 6 in]
  }
  "error out" <- w3
